vi "InverseModelForm.vi"() -> ()   [LabVIEW 2012]
panel:
  in  "ShowWeightedMean":bool caption="Weighted mean path"
  in  "ShowBestFit":bool caption="Best-fit model"
  in  "ShowSegLabel":bool caption="Segment labels"
  in  "Options":bool
  in  "Clear":bool
  in  "TestPath":bool
  in  "Terminate":bool
  in  "Start":bool
  in  "DisplayMode":string(combo) caption="Result to display:"
  in  "WatchItGo":bool caption="Watch it go?"
  in  "NumPaths":dbl caption="="
  in  "EndingCondition":string(combo) caption="Ending condition:"
  in  "Subsegment":string(combo) caption="Subsegment spacing:"
  in  "Method":string(combo) caption="Search method:"
  # "Show:"
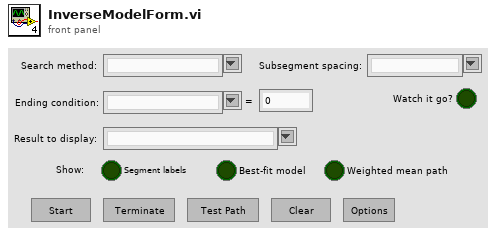
[diagram p1: front panel]
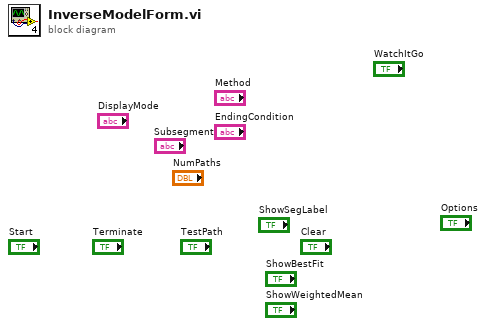
[diagram p0: block diagram]
diagram:
